vi "Create Cp plot.vi"(0 "Pressures in (cols = sensor, rows = time)":sgl[][](array[numeric])) -> (1 "Cp against x/c":cluster{"x/c flap (sorted)":sgl[], sgl[]}[](graph), 2 "Pdyn ref (Pa)":sgl)   [LabVIEW 2015]
panel:
  in  "Sensor index (sorted), flap":i32[](array[numeric])=[22, 23, 25, 26, 28, 29, 27, 24]
  in  "Sensor index (sorted), wing":i32[](array[numeric])=[2, 0, 13, 12, 11, 10, 6, 9, 5, 8, 7, 4, 21, 3, 20, 19, 18, 17, 16, 15, 14, 1]
  in  "Pdyn ref sensor no.":i32=32
  in  "x/c flap (sorted)":sgl[](array[numeric])=[0.9951131, 0.9789507, 0.94671166, 0.898568, 0.83493316, 0.80438995, 0.83493316, 0.9005628]
  in  "x/c wing (sorted)":sgl[](array[numeric])=[0.7367813, 0.48221973, 0.35498825, 0.23053746, 0.1323952, 0.06888126, 0.037189517, 0.029719163, 0.020091694, 0.008870252, 1.91e-05, 0.017702324, 0.027253436, 0.03684909, 0.046428833, 0.065556504, 0.08735989, 0.15782876, 0.28504115, 0.412279, 0.5395105, 0.6667451]
  # "Manually input and make default"
  # "Data sorted by winding no."
  # "Manually paste in data and then make default values"
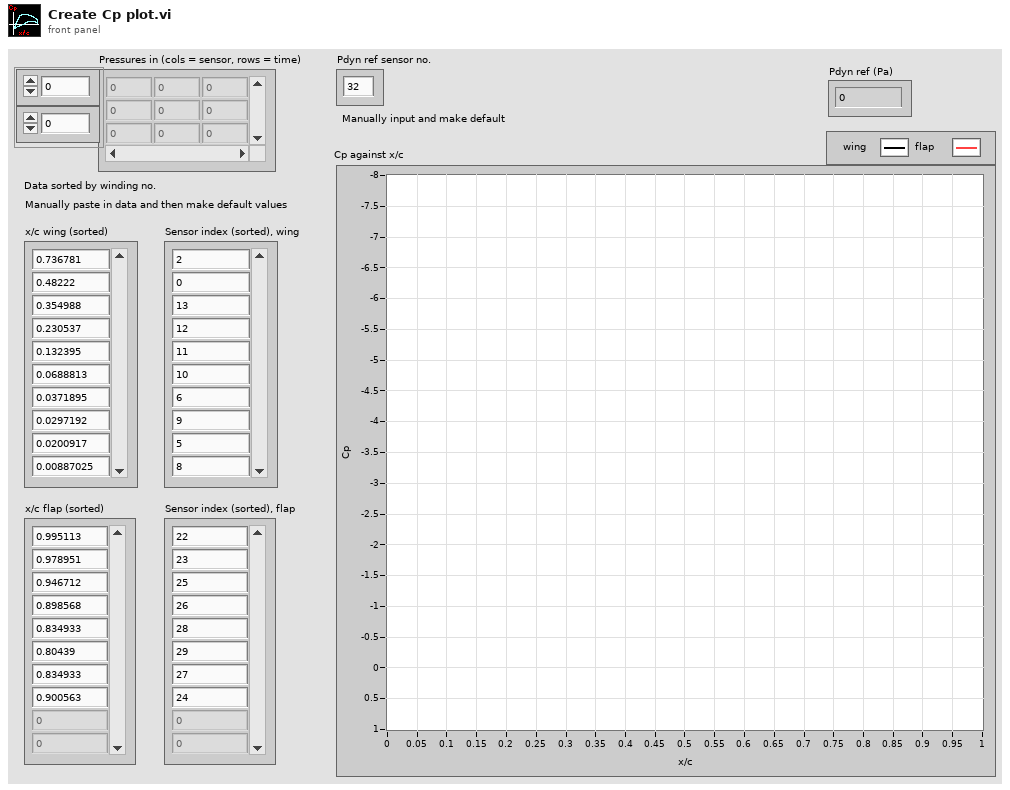
[diagram p1: front panel]
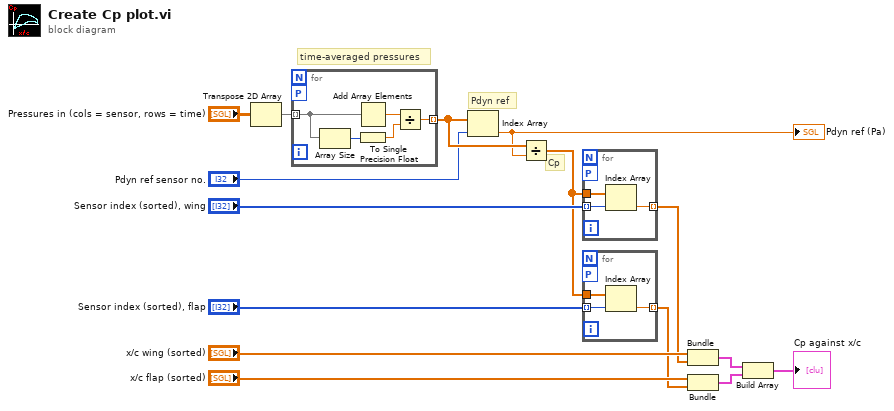
[diagram p0: block diagram]
diagram:
  # "Cp"
  # "Pdyn ref"
  # "time-averaged pressures"
  n1 = Transpose 2D Array(2D array="Pressures in (cols = sensor, rows = time)") -> (transposed array=w7:sgl[][])
  n2 = for {
    tunnel: w7 -> [w20] mode=indexing
    tunnel: [w16] -> w14 mode=indexing
    workers-P: _ -> [_]
    n3 = Array Size(array=w20) -> (size(s)=w18:i32)
    n4 = Add Array Elements(numeric array=w20) -> (sum=w19:sgl)
    n5 = To Single Precision Float(number=w18) -> (single precision float=w17:sgl)
    n6 = Divide(x=w19, y=w17) -> (x/y=w16:sgl)
  }
  n7 = Index Array(array=w14, index="Pdyn ref sensor no.") -> (element=w13:sgl)
  "Pdyn ref (Pa)" <- w13
  n8 = Divide(x=w14, y=w13) -> (x/y=w1:sgl[])
  n9 = for {
    tunnel: w1 -> [w23]
    tunnel: "Sensor index (sorted), wing" -> [w22] mode=indexing
    tunnel: [w21] -> w3 mode=indexing
    workers-P: _ -> [_]
    n10 = Index Array(array=w23, index=w22) -> (element=w21:sgl)
  }
  n11 = for {
    tunnel: w1 -> [w26]
    tunnel: "Sensor index (sorted), flap" -> [w25] mode=indexing
    tunnel: [w24] -> w2 mode=indexing
    workers-P: _ -> [_]
    n12 = Index Array(array=w26, index=w25) -> (element=w24:sgl)
  }
  n13 = Bundle("x/c wing (sorted)"="x/c wing (sorted)", w3) -> (w8:cluster{"x/c wing (sorted)":sgl[], sgl[]})  [unwired: 1 in]
  n14 = Bundle("x/c flap (sorted)"="x/c flap (sorted)", w2) -> (w12:cluster{"x/c flap (sorted)":sgl[], sgl[]})  [unwired: 1 in]
  n15 = Build Array(w8, w12) -> (→"Cp against x/c":cluster{"x/c flap (sorted)":sgl[], sgl[]}[])
